vi "StorageXMutationAddCloseTerm.vi"(1 "stateInfo out 2":T4) -> (0 "stateInfo out":T4)   [LabVIEW 2017]
uses:
  <vilib>/Platform/storage/lvStorage.llb/_stateInfoWriteProps.ctl
  <vilib>/Platform/storage/lvStorage.llb/dataStorageParams.ctl
  <vilib>/Platform/storage/lvStorage.llb/_selectedProp.ctl
  <vilib>/Platform/storage/lvStorage.llb/dataModel.ctl
  <vilib>/Platform/storage/Storage.llb/usiTypeDef.ctl
  <vilib>/Platform/storage/Storage.llb/usiPropDef.ctl
  <vilib>/express/express shared/ex_EditUserDefinedProperties/usiDataType.ctl
  <vilib>/Platform/storage/Storage.llb/specialProperties.ctl
  <vilib>/Platform/storage/Storage.llb/usiOverwriteOptions.ctl
  <vilib>/Platform/storage/lvStorage.llb/TerminalDef.ctl
  <vilib>/Platform/storage/lvStorage.llb/_TerminalStyle.ctl
  <vilib>/Utility/XNodeSupport.llb/XRect32.ctl
  <vilib>/Platform/storage/Storage.llb/usiSequenceRepresentation.ctl
  <vilib>/Platform/storage/lvStorage.llb/channelType.ctl
  <vilib>/Platform/storage/lvStorage.llb/_dataTerminals.ctl
  <vilib>/Platform/storage/lvStorage.llb/_dataTypeEnumForTerminals.ctl
panel:
  in  "terminalDef":T1={"direction"=enum."Input", "typeDescriptor"="", "color"=0, "oldTerm"=0, "style"=enum."Express", "optional"=FALSE, "bounds"={"t"=0, "l"=0, "b"=138, "r"=96}, "termRefs"=[], "Name"="", "Data"=variant, "wiredTypeDescriptor"=""}
  in  "Name":string="file path"
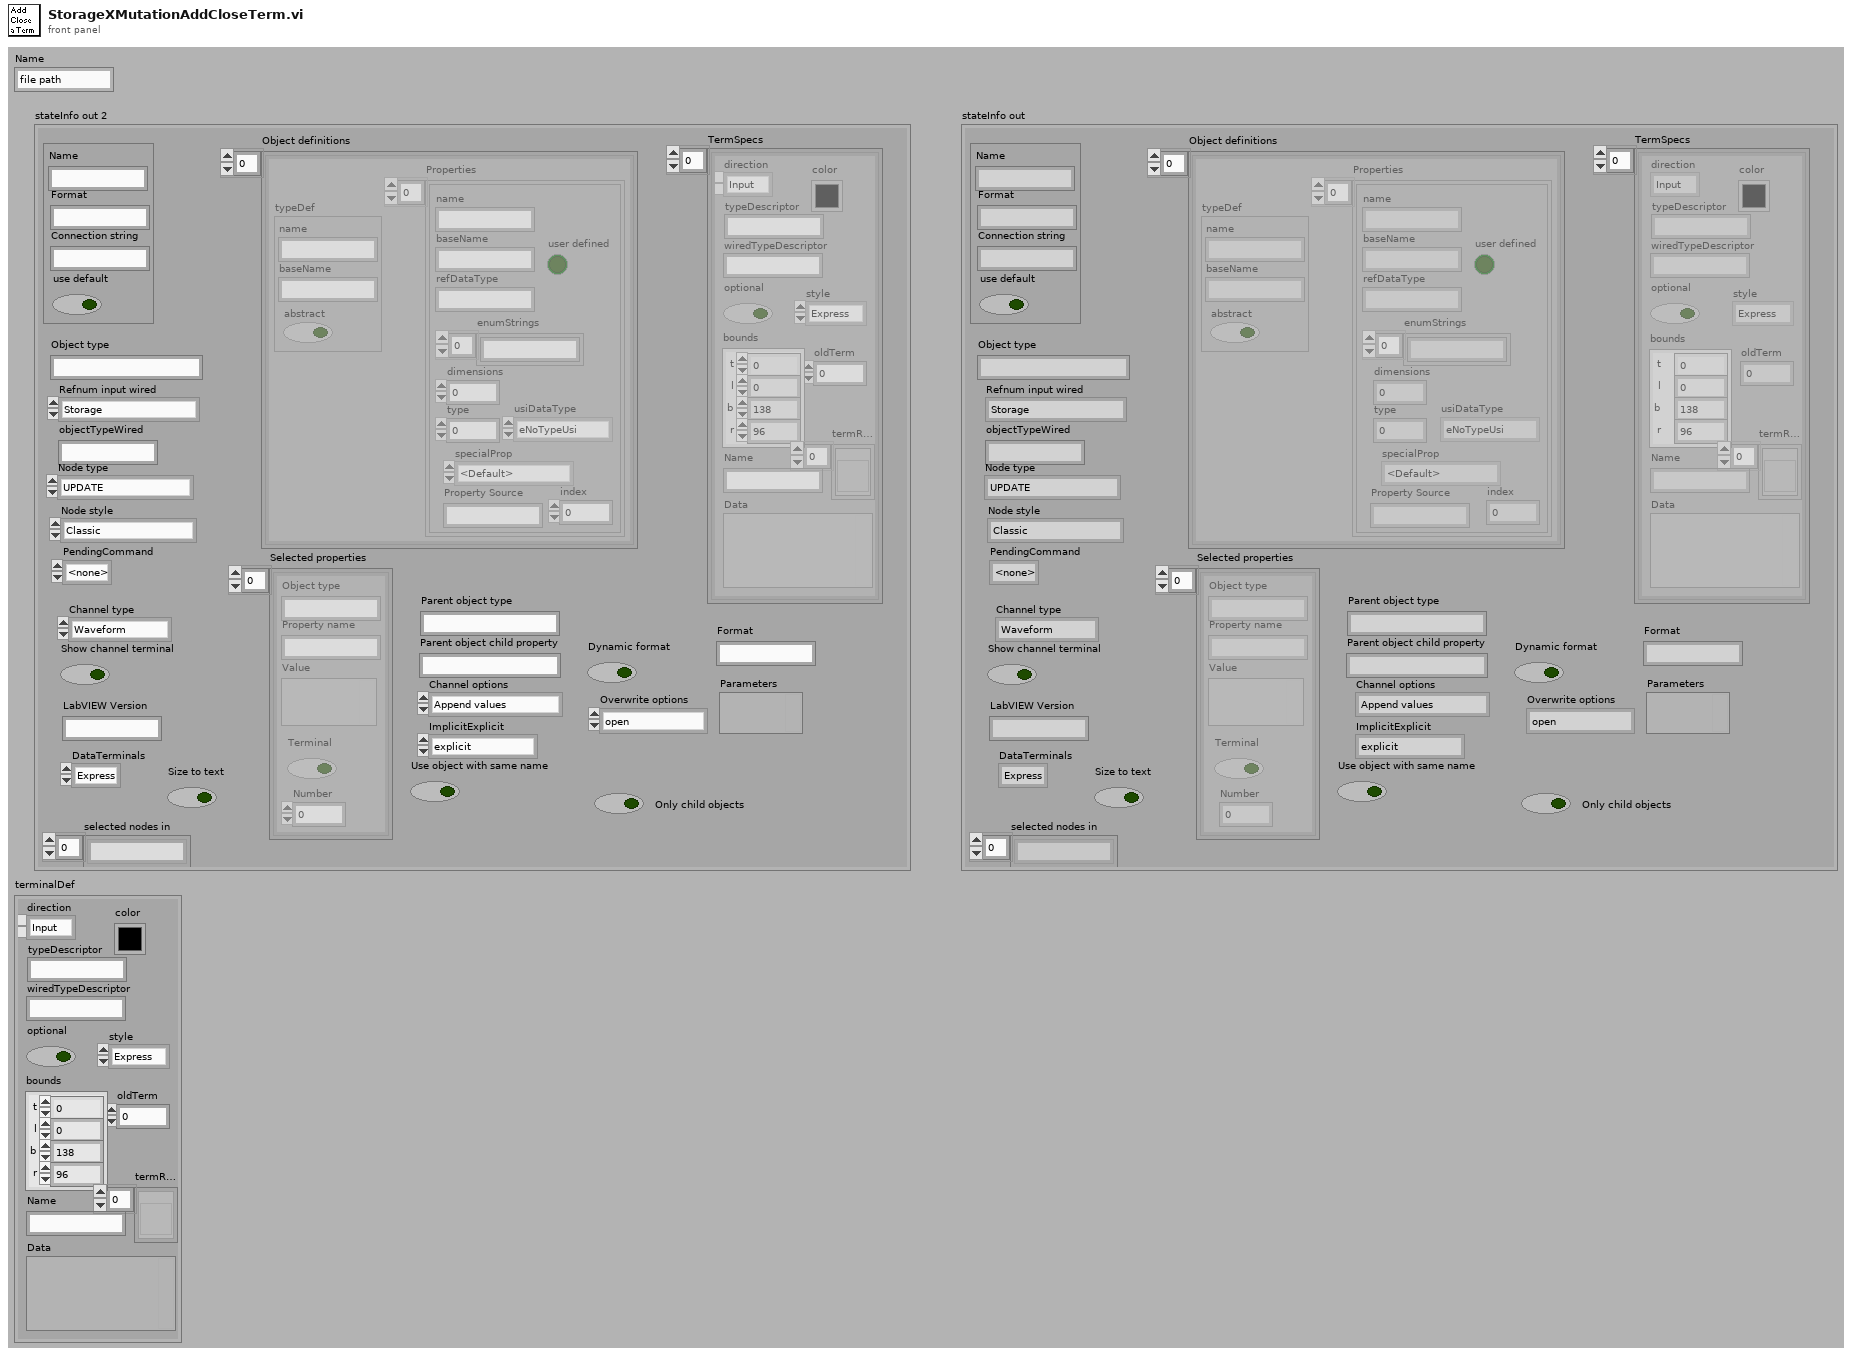
[diagram p1: front panel]
types:
  T1 = typedef "TerminalDef.ctl" = cluster{"direction":enum16{"Input", "Output"}, "typeDescriptor":string, "color":u32, "oldTerm":i32, "style":T2, "optional":bool, "bounds":T3, "termRefs":refnum<vi>[], "Name":string, "Data":variant, "wiredTypeDescriptor":string}
  T2 = typedef "_TerminalStyle.ctl" = enum16{"Express", "Collapsed", "Internal"}
  T3 = typedef "XRect32.ctl" = cluster{"t":i32, "l":i32, "b":i32, "r":i32}
  T4 = typedef "_stateInfoWriteProps.ctl" = cluster{"Data storage parameters":T5, "Object type":string, "Selected properties":T6[], "Object definitions":T7[], "Refnum input wired":enum16{"Storage", "Generic object", "Typed object", "<none>"}, "Parent object type":string, "Parent object child property":string, "Channel options":T12, "PendingCommand":enum16{"<none>", "SelPopUp", "Init"}, "Node style":enum16{"Classic", "Express"}, "Only child objects":bool, "TermSpecs":T1[], "objectTypeWired":string, "Dynamic format":bool, "Overwrite options":enum16{"open", "open or create", "create or replace", "create", "open (read only)"}, "Parameters":variant, "Format":string, "Node type":enum16{"UPDATE", "READ", "QUERY", "CREATE CHILD", "CREATE", "CONNECT", "DISCONNECT"}, "ImplicitExplicit":T13, "Channel type":T14, "Use object with same name":bool, "Show channel terminal":bool, "LabVIEW Version":string, "DataTerminals":T15, "Size to text":bool, "selected nodes in":string[]}
  T5 = typedef "dataStorageParams.ctl" = cluster{"Name":string, "Format":string, "Connection string":string, "use default":bool}
  T6 = typedef "_selectedProp.ctl" = cluster{"Object type":string, "Property name":string, "Value":variant, "Terminal":bool, "Number":i32}
  T7 = typedef "dataModel.ctl" = cluster{"typeDef":T8, "Properties":T9[]}
  T8 = typedef "usiTypeDef.ctl" = cluster{"name":string, "baseName":string, "abstract":bool}
  T9 = typedef "usiPropDef.ctl" = cluster{"name":string, "baseName":string, "refDataType":string, "dimensions":i32, "type":i32, "user defined":bool, "enumStrings":string[], "usiDataType":T10, "specialProp":T11, "Property Source":string, "index":i32}
  T10 = typedef "usiDataType.ctl" = enum16{"eNoTypeUsi", "eInt8Usi", "eInt16Usi", "eInt32Usi", "eInt64Usi", "eUInt8Usi", "eUInt16Usi", "eUInt32Usi", "eUInt64Usi", "eFloat32Usi", "eFloat64Usi", "- 0", "- 1", "- 2", "- 3", "- 4", "- 5", "- 6", "- 7", "- 8", "- 9", "eString8Usi", "eString16Usi", "eStringUsi", "eEnumUsi", "- 10", "- 11", "- 12", "- 13", "- 14", "eTimeUsi", "- 15", "- 16", "- 17", "- 18", "- 19", "- 20", "- 21", "- 22", "- 23", "eInstanceUsi", "eStoreUsi"}
  T11 = typedef "specialProperties.ctl" = enum16{"<Default>", "Channel Values", "AppendReplace", "ChannelFlags", "ValueFlags", "ImplicitExplicit", "InsertIndex", "ValuesCount", "ComparisonOperator", "Cluster", "DAQmx Channel"}
  T12 = typedef "usiOverwriteOptions.ctl" = enum16{"Append values", "Replace values at index", "Replace all values", "Append if timeline aligns"}
  T13 = typedef "usiSequenceRepresentation.ctl" = enum16{"explicit", "implicit"}
  T14 = typedef "channelType.ctl" = enum16{"Waveform", "Array of Double", "Array of String", "DDT", "Array of UInt8", "Array of Int16", "Array of Int32", "Array of Single", "Array of DateTime", "Array of Waveform", "none", "DateTime", "String", "Double", "Single", "UInt8", "Int16", "Int32"}
  T15 = typedef "_dataTerminals.ctl" = enum16{"Express", "Cluster"}
  T16 = enum16{"UPDATE", "READ", "QUERY", "CREATE CHILD", "CREATE", "CONNECT", "DISCONNECT"}
  T17 = typedef "_dataTypeEnumForTerminals.ctl" = enum16{"Data Storage", "Data Object", "Root", "Channel", "Error in", "Error out", "Storage Location (path)", "Storage Location (string)", "Storage Format", "Overwrite options (enum)", "Append / Replace (enum)", "index", "count", "Comparison (enum)", "Signal", "Channelgroup", "Cluster", "DBL", "SGL", "I32", "I16", "U8", "TIME", "STRING", "ENUM", "waveform", "DDT", "DAQmx Channel"}
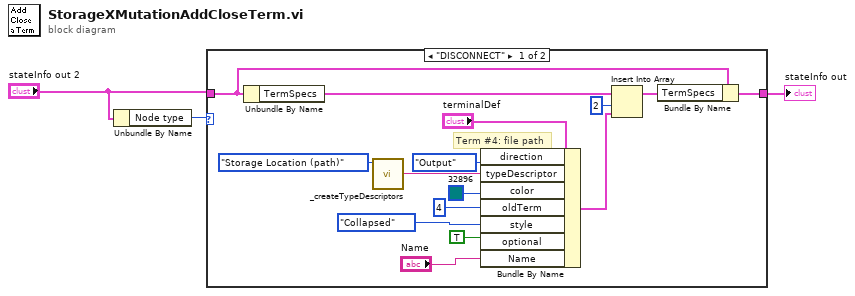
[diagram p0: block diagram]
diagram:
  n1 = Unbundle By Name("stateInfo out 2") -> ("Node type"=w1:T16)
  n2 = case shown="\"DISCONNECT\"" w1 {
    tunnel: "stateInfo out 2" -> [w6 w19]
    tunnel: [w4 w19] -> w3
    frame "DISCONNECT" {
      # "Term #4: file path"
      n3 = Unbundle By Name(w6) -> ("TermSpecs"=w9:T1[])
      n4 = call <vilib>:"_createTypeDescriptors.vi"("DNL_Data type"=_dataTypeEnumForTerminals."Storage Location (path)" ("Data type")) -> ("DNL_Type descriptor"=w14:string)  [unwired: 7 in, 3 out]
      n5 = Bundle By Name(cluster="terminalDef", "direction"=enum16{"Input", "Output"}."Output", "typeDescriptor"=w14, "color"=u32 32896 ("color(black)"), "oldTerm"=4, "style"=enum16{"Express", "Collapsed"}."Collapsed", "optional"=TRUE, "Name"="Name") -> (w7:T1)
      n6 = Insert Into Array(array=w9, index=2, new element=w7) -> (w5:T1[])
      n7 = Bundle By Name(cluster=w6, "TermSpecs"=w5) -> (w4:T4)
    }
    frame Default {
    }
  }
  "stateInfo out" <- w3
